vi "parseADCScanRateError.vi"(10 "ILCData in":T1 {"Responses"."ReportCalibrationData" items=["OK"=0, "IllegalFunction"=1, "IllegalDataAddress"=2, "IllegalDataValue"=3, "SlaveDeviceFailure"=4, "Acknowledge"=5, "SlaveDeviceBusy"=6, "NegativeAcknowledge"=7, "MemoryParityError"=8, "GatewayPathUnavailable"=9, "GatewayTargetDeviceFailedToRespond"=10, "WaitingForResponse"=254, "CRCError"=255]; "Responses"."ADCOffsetSensitivity" items=["OK"=0, "IllegalFunction"=1, "IllegalDataAddress"=2, "IllegalDataValue"=3, "SlaveDeviceFailure"=4, "Acknowledge"=5, "SlaveDeviceBusy"=6, "NegativeAcknowledge"=7, "MemoryParityError"=8, "GatewayPathUnavailable"=9, "GatewayTargetDeviceFailedToRespond"=10, "WaitingForResponse"=254, "CRCError"=255]; "Responses"."ADCScanRate" items=["OK"=0, "IllegalFunction"=1, "IllegalDataAddress"=2, "IllegalDataValue"=3, "SlaveDeviceFailure"=4, "Acknowledge"=5, "SlaveDeviceBusy"=6, "NegativeAcknowledge"=7, "MemoryParityError"=8, "GatewayPathUnavailable"=9, "GatewayTargetDeviceFailedToRespond"=10, "WaitingForResponse"=254, "CRCError"=255]; "Responses"."Reset" items=["OK"=0, "IllegalFunction"=1, "IllegalDataAddress"=2, "IllegalDataValue"=3, "SlaveDeviceFailure"=4, "Acknowledge"=5, "SlaveDeviceBusy"=6, "NegativeAcknowledge"=7, "MemoryParityError"=8, "GatewayPathUnavailable"=9, "GatewayTargetDeviceFailedToRespond"=10, "WaitingForResponse"=254, "CRCError"=255]; "Responses"."TemporaryAddress" items=["OK"=0, "IllegalFunction"=1, "IllegalDataAddress"=2, "IllegalDataValue"=3, "SlaveDeviceFailure"=4, "Acknowledge"=5, "SlaveDeviceBusy"=6, "NegativeAcknowledge"=7, "MemoryParityError"=8, "GatewayPathUnavailable"=9, "GatewayTargetDeviceFailedToRespond"=10, "WaitingForResponse"=254, "CRCError"=255]; "Responses"."Mode" items=["OK"=0, "IllegalFunction"=1, "IllegalDataAddress"=2, "IllegalDataValue"=3, "SlaveDeviceFailure"=4, "Acknowledge"=5, "SlaveDeviceBusy"=6, "NegativeAcknowledge"=7, "MemoryParityError"=8, "GatewayPathUnavailable"=9, "GatewayTargetDeviceFailedToRespond"=10, "WaitingForResponse"=254, "CRCError"=255]; "Responses"."ReportServerStatus" items=["OK"=0, "IllegalFunction"=1, "IllegalDataAddress"=2, "IllegalDataValue"=3, "SlaveDeviceFailure"=4, "Acknowledge"=5, "SlaveDeviceBusy"=6, "NegativeAcknowledge"=7, "MemoryParityError"=8, "GatewayPathUnavailable"=9, "GatewayTargetDeviceFailedToRespond"=10, "WaitingForResponse"=254, "CRCError"=255]; "Responses"."ReportServerID" items=["OK"=0, "IllegalFunction"=1, "IllegalDataAddress"=2, "IllegalDataValue"=3, "SlaveDeviceFailure"=4, "Acknowledge"=5, "SlaveDeviceBusy"=6, "NegativeAcknowledge"=7, "MemoryParityError"=8, "GatewayPathUnavailable"=9, "GatewayTargetDeviceFailedToRespond"=10, "WaitingForResponse"=254, "CRCError"=255]; "Telemetry"."ADCScanRate" items=["50 Hz"=0, "60 Hz"=1, "100 Hz"=2, "120 Hz"=3, "200 Hz"=4, "240 Hz"=5, "300 Hz"=6, "400 Hz"=7, "480 Hz"=8, "600 Hz"=9, "1200 Hz"=10, "2400 Hz"=11, "4800 Hz"=12, "No Change"=255]; "Command"."ADCScanRate" items=["50 Hz"=0, "60 Hz"=1, "100 Hz"=2, "120 Hz"=3, "200 Hz"=4, "240 Hz"=5, "300 Hz"=6, "400 Hz"=7, "480 Hz"=8, "600 Hz"=9, "1200 Hz"=10, "2400 Hz"=11, "4800 Hz"=12, "No Change"=255]}, 11 "ModbusBuffer in":T10) -> (2 "ILCData out":T1 {"Responses"."ReportCalibrationData" items=["OK"=0, "IllegalFunction"=1, "IllegalDataAddress"=2, "IllegalDataValue"=3, "SlaveDeviceFailure"=4, "Acknowledge"=5, "SlaveDeviceBusy"=6, "NegativeAcknowledge"=7, "MemoryParityError"=8, "GatewayPathUnavailable"=9, "GatewayTargetDeviceFailedToRespond"=10, "WaitingForResponse"=254, "CRCError"=255]; "Responses"."ADCOffsetSensitivity" items=["OK"=0, "IllegalFunction"=1, "IllegalDataAddress"=2, "IllegalDataValue"=3, "SlaveDeviceFailure"=4, "Acknowledge"=5, "SlaveDeviceBusy"=6, "NegativeAcknowledge"=7, "MemoryParityError"=8, "GatewayPathUnavailable"=9, "GatewayTargetDeviceFailedToRespond"=10, "WaitingForResponse"=254, "CRCError"=255]; "Responses"."ADCScanRate" items=["OK"=0, "IllegalFunction"=1, "IllegalDataAddress"=2, "IllegalDataValue"=3, "SlaveDeviceFailure"=4, "Acknowledge"=5, "SlaveDeviceBusy"=6, "NegativeAcknowledge"=7, "MemoryParityError"=8, "GatewayPathUnavailable"=9, "GatewayTargetDeviceFailedToRespond"=10, "WaitingForResponse"=254, "CRCError"=255]; "Responses"."Reset" items=["OK"=0, "IllegalFunction"=1, "IllegalDataAddress"=2, "IllegalDataValue"=3, "SlaveDeviceFailure"=4, "Acknowledge"=5, "SlaveDeviceBusy"=6, "NegativeAcknowledge"=7, "MemoryParityError"=8, "GatewayPathUnavailable"=9, "GatewayTargetDeviceFailedToRespond"=10, "WaitingForResponse"=254, "CRCError"=255]; "Responses"."TemporaryAddress" items=["OK"=0, "IllegalFunction"=1, "IllegalDataAddress"=2, "IllegalDataValue"=3, "SlaveDeviceFailure"=4, "Acknowledge"=5, "SlaveDeviceBusy"=6, "NegativeAcknowledge"=7, "MemoryParityError"=8, "GatewayPathUnavailable"=9, "GatewayTargetDeviceFailedToRespond"=10, "WaitingForResponse"=254, "CRCError"=255]; "Responses"."Mode" items=["OK"=0, "IllegalFunction"=1, "IllegalDataAddress"=2, "IllegalDataValue"=3, "SlaveDeviceFailure"=4, "Acknowledge"=5, "SlaveDeviceBusy"=6, "NegativeAcknowledge"=7, "MemoryParityError"=8, "GatewayPathUnavailable"=9, "GatewayTargetDeviceFailedToRespond"=10, "WaitingForResponse"=254, "CRCError"=255]; "Responses"."ReportServerStatus" items=["OK"=0, "IllegalFunction"=1, "IllegalDataAddress"=2, "IllegalDataValue"=3, "SlaveDeviceFailure"=4, "Acknowledge"=5, "SlaveDeviceBusy"=6, "NegativeAcknowledge"=7, "MemoryParityError"=8, "GatewayPathUnavailable"=9, "GatewayTargetDeviceFailedToRespond"=10, "WaitingForResponse"=254, "CRCError"=255]; "Responses"."ReportServerID" items=["OK"=0, "IllegalFunction"=1, "IllegalDataAddress"=2, "IllegalDataValue"=3, "SlaveDeviceFailure"=4, "Acknowledge"=5, "SlaveDeviceBusy"=6, "NegativeAcknowledge"=7, "MemoryParityError"=8, "GatewayPathUnavailable"=9, "GatewayTargetDeviceFailedToRespond"=10, "WaitingForResponse"=254, "CRCError"=255]; "Telemetry"."ADCScanRate" items=["50 Hz"=0, "60 Hz"=1, "100 Hz"=2, "120 Hz"=3, "200 Hz"=4, "240 Hz"=5, "300 Hz"=6, "400 Hz"=7, "480 Hz"=8, "600 Hz"=9, "1200 Hz"=10, "2400 Hz"=11, "4800 Hz"=12, "No Change"=255]; "Command"."ADCScanRate" items=["50 Hz"=0, "60 Hz"=1, "100 Hz"=2, "120 Hz"=3, "200 Hz"=4, "240 Hz"=5, "300 Hz"=6, "400 Hz"=7, "480 Hz"=8, "600 Hz"=9, "1200 Hz"=10, "2400 Hz"=11, "4800 Hz"=12, "No Change"=255]}, 3 "ModbusBuffer out":T10)   [LabVIEW 2016]
uses:
  Utilities/Modbus/DataTypes/ModbusBuffer.ctl
  DataTypes/ILCData.ctl
  DataTypes/ILCConstants.ctl
  DataTypes/ILCCommand.ctl
  DataTypes/ILCScanRates.ctl
  DataTypes/ILCTelemetry.ctl
  DataTypes/ILCResponses.ctl
  Common_RT_Modbus/DataTypes/ExceptionCodes.ctl
  DataTypes/ILCTimestamps.ctl
  DataTypes/ILCTimings.ctl
  Common_RT_Modbus/RTModbus.lvlib
  Utilities/Modbus/ModbusUtilities.lvlib
  RTILC.lvlib
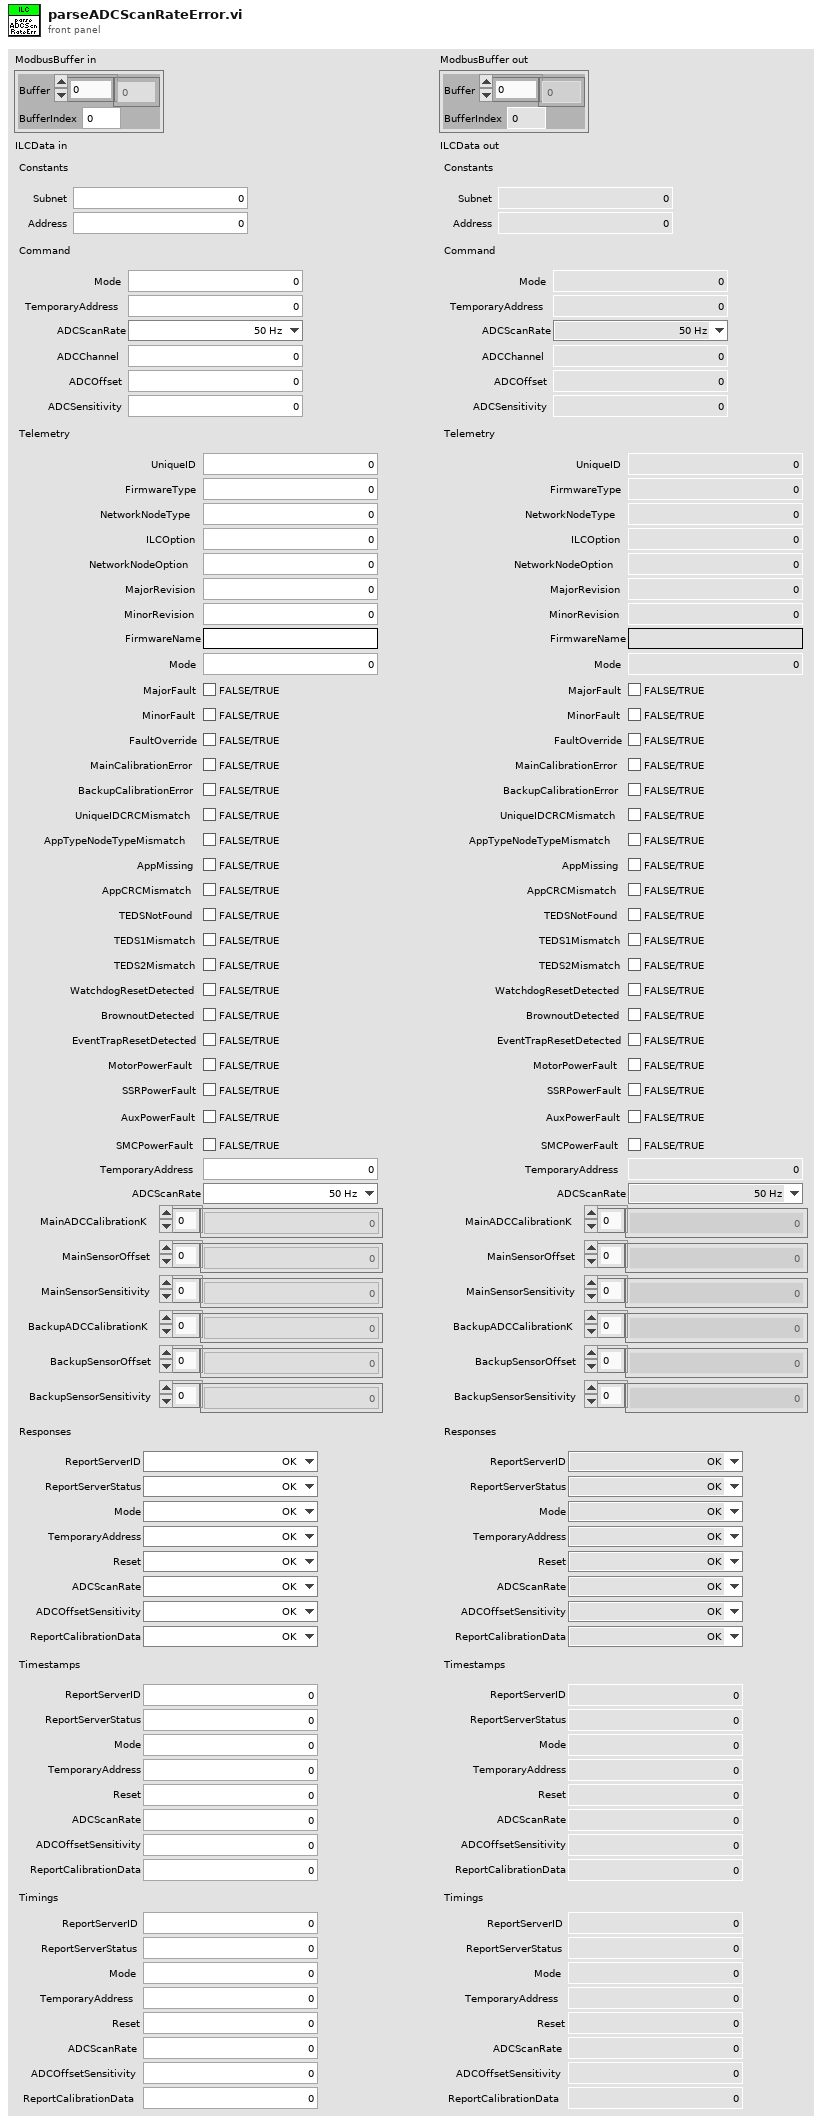
[diagram p1: front panel]
types:
  T1 = typedef "RTILC.lvlib/ILCData.ctl" = cluster{"Constants":T2, "Command":T3, "Telemetry":T5, "Responses":T6, "Timestamps":T8, "Timings":T9}
  T2 = typedef "RTILC.lvlib/ILCConstants.ctl" = cluster{"Subnet":u8, "Address":u8}
  T3 = typedef "RTILC.lvlib/ILCCommand.ctl" = cluster{"Mode":u16, "TemporaryAddress":u8, "ADCScanRate":T4, "ADCChannel":u8, "ADCOffset":sgl, "ADCSensitivity":sgl}
  T4 = typedef "RTILC.lvlib/ILCScanRates.ctl" = u8
  T5 = typedef "RTILC.lvlib/ILCTelemetry.ctl" = cluster{"UniqueID":u64, "FirmwareType":u8, "NetworkNodeType":u8, "ILCOption":u8, "NetworkNodeOption":u8, "MajorRevision":u8, "MinorRevision":u8, "FirmwareName":string, "Mode":u16, "MajorFault":bool, "MinorFault":bool, "FaultOverride":bool, "MainCalibrationError":bool, "BackupCalibrationError":bool, "UniqueIDCRCMismatch":bool, "AppTypeNodeTypeMismatch":bool, "AppMissing":bool, "AppCRCMismatch":bool, "TEDSNotFound":bool, "TEDS1Mismatch":bool, "TEDS2Mismatch":bool, "WatchdogResetDetected":bool, "BrownoutDetected":bool, "EventTrapResetDetected":bool, "MotorPowerFault":bool, "SSRPowerFault":bool, "AuxPowerFault":bool, "SMCPowerFault":bool, "TemporaryAddress":u8, "ADCScanRate":T4, "MainADCCalibrationK":sgl[], "MainSensorOffset":sgl[], "MainSensorSensitivity":sgl[], "BackupADCCalibrationK":sgl[], "BackupSensorOffset":sgl[], "BackupSensorSensitivity":sgl[]}
  T6 = typedef "RTILC.lvlib/ILCResponses.ctl" = cluster{"ReportServerID":T7, "ReportServerStatus":T7, "Mode":T7, "TemporaryAddress":T7, "Reset":T7, "ADCScanRate":T7, "ADCOffsetSensitivity":T7, "ReportCalibrationData":T7}
  T7 = typedef "RTModbus.lvlib/ExceptionCodes.ctl" = u16
  T8 = typedef "RTILC.lvlib/ILCTimestamps.ctl" = cluster{"ReportServerID":dbl, "ReportServerStatus":dbl, "Mode":dbl, "TemporaryAddress":dbl, "Reset":dbl, "ADCScanRate":dbl, "ADCOffsetSensitivity":dbl, "ReportCalibrationData":dbl}
  T9 = typedef "RTILC.lvlib/ILCTimings.ctl" = cluster{"ReportServerID":u32, "ReportServerStatus":u32, "Mode":u32, "TemporaryAddress":u32, "Reset":u32, "ADCScanRate":u32, "ADCOffsetSensitivity":u32, "ReportCalibrationData":u32}
  T10 = typedef "ModbusUtilities.lvlib/ModbusBuffer.ctl" = cluster{"Buffer":u16[], "BufferIndex":i32}
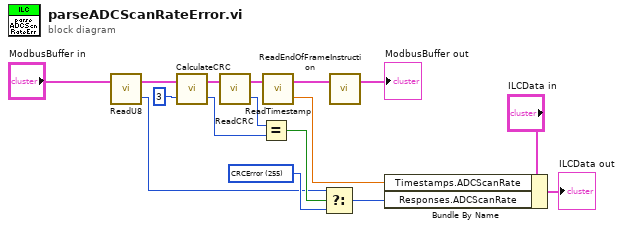
[diagram p0: block diagram]
diagram:
  w6 = T7 255 items=["OK"=0, "IllegalFunction"=1, "IllegalDataAddress"=2, "IllegalDataValue"=3, "SlaveDeviceFailure"=4, "Acknowledge"=5, "SlaveDeviceBusy"=6, "NegativeAcknowledge"=7, "MemoryParityError"=8, "GatewayPathUnavailable"=9, "GatewayTargetDeviceFailedToRespond"=10, "WaitingForResponse"=254, "CRCError"=255] ("f")
  n1 = call "ReadU8.vi"("ModbusBuffer in"="ModbusBuffer in") -> ("Output"=w1:u8, "ModbusBuffer out"=w2:T10)  [unwired: 1 in]
  n2 = call "CalculateCRC.vi"("Length"=3, "ModbusBuffer in"=w2) -> ("CRC"=w8:u16, "ModbusBuffer out"=w11:T10)
  n3 = call "ReadCRC.vi"("ModbusBuffer in"=w11) -> ("CRC"=w9:u16, "ModbusBuffer out"=w14:T10)  [unwired: 1 in]
  n4 = Equal?(x=w9, y=w8) -> (x = y?=w7:bool)
  n5 = call "ReadTimestamp.vi"("ModbusBuffer in"=w14) -> ("Output"=w4:dbl, "ModbusBuffer out"=w13:T10)  [unwired: 1 in]
  n6 = Select(t=w1, s=w7, f=w6) -> (s? t:f=w5:T7)
  n7 = call "ReadEndOfFrameInstruction.vi"("ModbusBuffer in"=w13) -> ("ModbusBuffer out"=→"ModbusBuffer out":T10)  [unwired: 2 in]
  n8 = Bundle By Name(cluster="ILCData in", "Timestamps.ADCScanRate"=w4, "Responses.ADCScanRate"=w5) -> (→"ILCData out":T1)
